vi "Lift.vi"(10 "lift":dbl) -> ()   [LabVIEW 2014]
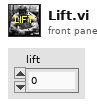
[diagram p1: front panel]
types:
  T1 = typedef "WPI_DigitalInputDevRef.ctl" = cluster{"DevStatus":errorcluster, "DIO Channel":T2, "Controller":T3}
  T2 = typedef "FPGA_DIOChannel.ctl" = enum8{"DIO 0", "DIO 1", "DIO 2", "DIO 3", "DIO 4", "DIO 5", "DIO 6", "DIO 7", "DIO 8", "DIO 9", "DIO MXP 0", "DIO MXP 1", "DIO MXP 2", "DIO MXP 3", "DIO MXP 4", "DIO MXP 5", "DIO MXP 6", "DIO MXP 7", "DIO MXP 8", "DIO MXP 9", "DIO MXP 10", "DIO MXP 11", "DIO MXP 12", "DIO MXP 13", "DIO MXP 14", "DIO MXP 15", "Invalid"}
  T3 = typedef "FPGA_TypedefDigitalModule.ctl" = enum16{"Controller 1"}
  T4 = typedef "WPI_EncoderDevRef.ctl" = cluster{"DevStatus":errorcluster, "EncoderIndex":T5, "CounterIndex":T6, "DistancePerCount":dbl, "Decoding Type":T7}
  T5 = typedef "FPGA_EncoderIdx.ctl" = enum8{"Enc 0", "Enc 1", "Enc 2", "Enc 3", "Enc 4", "Enc 5", "Enc 6", "Enc 7", "Invalid"}
  T6 = typedef "FPGA_CounterCtrSystemIndex.ctl" = enum8{"Ctr 0", "Ctr 1", "Ctr 2", "Ctr 3", "Ctr 4", "Ctr 5", "Ctr 6", "Ctr 7", "Invalid"}
  T7 = typedef "WPI_EncoderType.ctl" = enum16{"1x", "2x", "4x"}
  T8 = typedef "WPI_MotorControlDeviceRef.ctl" = cluster{"DeviceStatus":errorcluster, "Type":T9, "PWM":cluster{"Controller":T3, "PWM Channel":T10, "DeadBand":T11}, "CAN":cluster{"Device Number":u8, "Control Mode":T12, "Semaphore":T13, "Max Vout":dbl, "TalonSRX Control Mode":T14}, "Invert":bool, "TransformRef":T15, "InvTransformRef":T15}
  T9 = typedef "WPI_MotorControlType.ctl" = enum16{"PWM", "CAN", "CANTalonSRX"}
  T10 = typedef "FPGA_DIOPWMChannel.ctl" = enum8{"PWM 0", "PWM 1", "PWM 2", "PWM 3", "PWM 4", "PWM 5", "PWM 6", "PWM 7", "PWM 8", "PWM 9", "PWM MXP 0", "PWM MXP 1", "PWM MXP 2", "PWM MXP 3", "PWM MXP 4", "PWM MXP 5", "PWM MXP 6", "PWM MXP 7", "PWM MXP 8", "PWM MXP 9", "Invalid"}
  T11 = typedef "WPI_PWMDeadband.ctl" = cluster{"Name":string, "maxPositivePwm":i32, "minPositivePwm":i32, "centerPwm":i32, "maxNegativePwm":i32, "minNegativePwm":i32, "angularRange":u16}
  T12 = typedef "WPI_CANJaguar_ControlMode.ctl" = enum8{"Percent VBus", "Current", "Speed", "Position", "Voltage"}
  T13 = typedef "Semaphore RefNum" = refnum<k1>
  T14 = typedef "WPI_CANTalonSRX_APIControlMode.ctl" = enum8{"Percent VBus", "Speed", "Position", "Slave", "Unchanged / Invalid"}
  T15 = typedef "WPI_PWMTransform_ConPane.ctl" = refnum<vi>
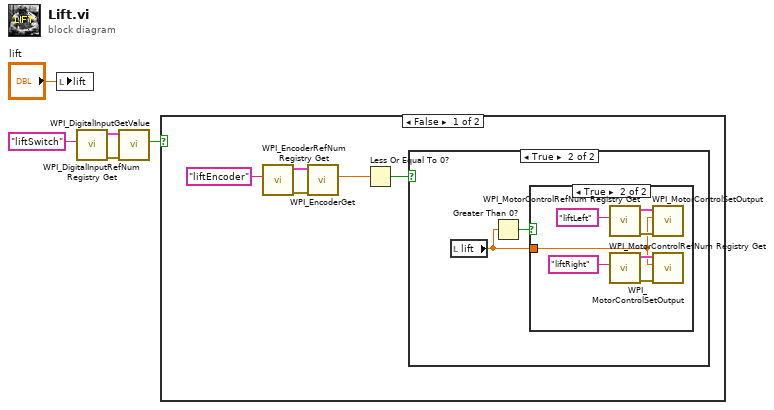
[diagram p0: block diagram]
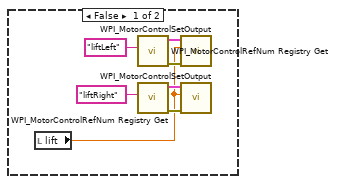
[diagram p2: hidden frame]
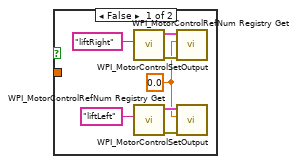
[diagram p3: hidden frame]
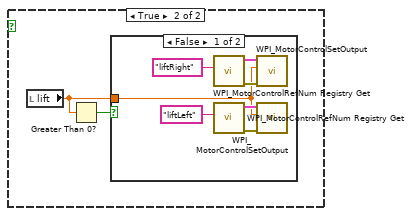
[diagram p4: hidden frame]
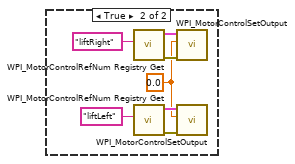
[diagram p5: hidden frame]
diagram:
  n1 = local write "lift"("lift") -> ()
  n2 = call <vilib>:"WPI_DigitalInputRefNum Registry Get.vi"("refnum name"="liftSwitch") -> ("error out"=w4:errorcluster, "DigitalInputDevRef"=w3:T1)  [unwired: 9 in]
  n3 = call <vilib>:"WPI_DigitalInputGetValue.vi"("error in (no error)"=w4, "DigitalInputDevRef"=w3) -> ("Value"=w1:bool)  [unwired: 7 in, 2 out]
  n4 = case shown="False" w1 {
    frame False {
      n5 = call <vilib>:"WPI_EncoderRefNum Registry Get.vi"("refnum name"="liftEncoder") -> ("error out"=w10:errorcluster, "EncoderDevRef"=w9:T4)  [unwired: 9 in]
      n6 = call <vilib>:"WPI_EncoderGet.vi"("error in (no error)"=w10, "EncoderDevRef"=w9) -> ("Distance"=w7:dbl)  [unwired: 4 in, 5 out]
      n7 = Less Or Equal To 0?(x=w7) -> (x <= 0?=w6:bool)
      n8 = case shown="True" w6 {
        frame False {
          n9 = local read "lift"() -> (w11:dbl)
          n10 = call <vilib>:"WPI_MotorControlRefNum Registry Get.vi"("refnum name"="liftLeft") -> ("error out"=w12:errorcluster, "MotorControlDevRef"=w17:T8)  [unwired: 9 in]
          n11 = call <vilib>:"WPI_MotorControlRefNum Registry Get.vi"("refnum name"="liftRight") -> ("error out"=w15:errorcluster, "MotorControlDevRef"=w13:T8)  [unwired: 9 in]
          n12 = call <vilib>:"WPI_MotorControlSetOutput.vi"("error in (no error)"=w12, "Output"=w11, "MotorControlDevRef"=w17) -> ()  [unwired: 6 in, 3 out]
          n13 = call <vilib>:"WPI_MotorControlSetOutput.vi"("error in (no error)"=w15, "Output"=w11, "MotorControlDevRef"=w13) -> ()  [unwired: 6 in, 3 out]
        }
        frame True {
          n14 = local read "lift"() -> (w18:dbl)
          n15 = Greater Than 0?(x=w18) -> (x > 0?=w19:bool)
          n16 = case shown="True" w19 {
            tunnel: w18 -> [_ w27]
            frame False {
              w20 = 0.0 ("Output")
              n17 = call <vilib>:"WPI_MotorControlRefNum Registry Get.vi"("refnum name"="liftRight") -> ("error out"=w24:errorcluster, "MotorControlDevRef"=w22:T8)  [unwired: 9 in]
              n18 = call <vilib>:"WPI_MotorControlRefNum Registry Get.vi"("refnum name"="liftLeft") -> ("error out"=w21:errorcluster, "MotorControlDevRef"=w26:T8)  [unwired: 9 in]
              n19 = call <vilib>:"WPI_MotorControlSetOutput.vi"("error in (no error)"=w24, "Output"=w20, "MotorControlDevRef"=w22) -> ()  [unwired: 6 in, 3 out]
              n20 = call <vilib>:"WPI_MotorControlSetOutput.vi"("error in (no error)"=w21, "Output"=w20, "MotorControlDevRef"=w26) -> ()  [unwired: 6 in, 3 out]
            }
            frame True {
              n21 = call <vilib>:"WPI_MotorControlRefNum Registry Get.vi"("refnum name"="liftLeft") -> ("error out"=w28:errorcluster, "MotorControlDevRef"=w33:T8)  [unwired: 9 in]
              n22 = call <vilib>:"WPI_MotorControlRefNum Registry Get.vi"("refnum name"="liftRight") -> ("error out"=w31:errorcluster, "MotorControlDevRef"=w29:T8)  [unwired: 9 in]
              n23 = call <vilib>:"WPI_MotorControlSetOutput.vi"("error in (no error)"=w28, "Output"=w27, "MotorControlDevRef"=w33) -> ()  [unwired: 6 in, 3 out]
              n24 = call <vilib>:"WPI_MotorControlSetOutput.vi"("error in (no error)"=w31, "Output"=w27, "MotorControlDevRef"=w29) -> ()  [unwired: 6 in, 3 out]
            }
          }
        }
      }
    }
    frame True {
      n25 = local read "lift"() -> (w34:dbl)
      n26 = Greater Than 0?(x=w34) -> (x > 0?=w35:bool)
      n27 = case shown="False" w35 {
        tunnel: w34 -> [w36 _]
        frame False {
          n28 = call <vilib>:"WPI_MotorControlRefNum Registry Get.vi"("refnum name"="liftRight") -> ("error out"=w40:errorcluster, "MotorControlDevRef"=w38:T8)  [unwired: 9 in]
          n29 = call <vilib>:"WPI_MotorControlRefNum Registry Get.vi"("refnum name"="liftLeft") -> ("error out"=w37:errorcluster, "MotorControlDevRef"=w42:T8)  [unwired: 9 in]
          n30 = call <vilib>:"WPI_MotorControlSetOutput.vi"("error in (no error)"=w40, "Output"=w36, "MotorControlDevRef"=w38) -> ()  [unwired: 6 in, 3 out]
          n31 = call <vilib>:"WPI_MotorControlSetOutput.vi"("error in (no error)"=w37, "Output"=w36, "MotorControlDevRef"=w42) -> ()  [unwired: 6 in, 3 out]
        }
        frame True {
          w43 = 0.0 ("Output")
          n32 = call <vilib>:"WPI_MotorControlRefNum Registry Get.vi"("refnum name"="liftRight") -> ("error out"=w47:errorcluster, "MotorControlDevRef"=w45:T8)  [unwired: 9 in]
          n33 = call <vilib>:"WPI_MotorControlRefNum Registry Get.vi"("refnum name"="liftLeft") -> ("error out"=w44:errorcluster, "MotorControlDevRef"=w49:T8)  [unwired: 9 in]
          n34 = call <vilib>:"WPI_MotorControlSetOutput.vi"("error in (no error)"=w47, "Output"=w43, "MotorControlDevRef"=w45) -> ()  [unwired: 6 in, 3 out]
          n35 = call <vilib>:"WPI_MotorControlSetOutput.vi"("error in (no error)"=w44, "Output"=w43, "MotorControlDevRef"=w49) -> ()  [unwired: 6 in, 3 out]
        }
      }
    }
  }
